vi "Configure.vi"(6 "Setpoint Range":cluster{"Max":dbl, "Min":dbl}, 7 "Process Span":cluster{"Max":dbl, "Min":dbl}, 8 "error in (no error)":errorcluster, 9 "Output Range":cluster{"Max":dbl, "Min":dbl}, 10 "PID Gains":cluster{"Kp":dbl, "Ki":dbl, "Kd":dbl}, 11 "PID in":refnum<class "PID.lvclass">) -> (0 "error out":errorcluster, 3 "PID out":refnum<class "PID.lvclass">)   [LabVIEW 2025, in "PID.lvlib" / "PID.lvclass"]
uses:
  PID.lvclass
  PID.lvclass/PID.ctl
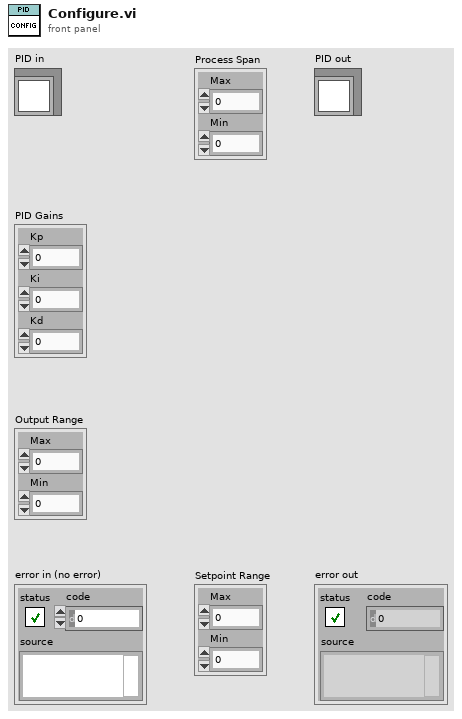
[diagram p1: front panel]
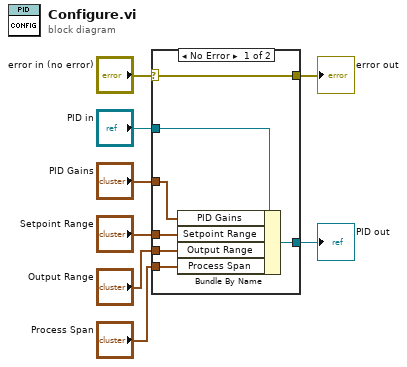
[diagram p0: block diagram]
diagram:
  n1 = case shown="No Error" "error in (no error)" {
    selector: "error in (no error)" -> [w15 w17]
    tunnel: [w15 w17] -> w7
    tunnel: [w13 w16] -> w5
    tunnel: "PID in" -> [w14 w16]
    tunnel: "PID Gains" -> [w12 _]
    tunnel: "Setpoint Range" -> [w11 _]
    tunnel: "Output Range" -> [w10 _]
    tunnel: "Process Span" -> [w9 _]
    frame No Error {
      n2 = Bundle By Name(cluster=w14, "PID Gains"=w12, "Setpoint Range"=w11, "Output Range"=w10, "Process Span"=w9) -> (w13:refnum<class "PID.lvclass">)
    }
    frame Error {
    }
  }
  "error out" <- w7
  "PID out" <- w5
